vi "V7310.Main.Init.vi"(8 "error in":errorcluster, 11 "Data in":T1={"Status"={"State"=enum."Init", "LaserStatus"=enum."-", "LaserStatusRaw"="", "Ref"=refnum, "RTC TS"=timestamp(0 s since 1904-01-01), "Conn TS"=timestamp(0 s since 1904-01-01), "Msg"=[], "JobInUse"="", "Jobs"=[], "Vars"=[]}, "Sets"={"Address"="192.168.2.1", "Timeout_ms"=5000, "ReconnectPeriod_s"=0, "JobInUse"="", "CoordinatesOffset"={"X"=0.0, "Y"=0.0}}}) -> (0 "error out":errorcluster, 3 "Data out":T1={"Status"={"State"=enum."Init", "LaserStatus"=enum."-", "LaserStatusRaw"="", "Ref"=refnum, "RTC TS"=timestamp(0 s since 1904-01-01), "Conn TS"=timestamp(0 s since 1904-01-01), "Msg"=[], "JobInUse"="", "Jobs"=[], "Vars"=[]}, "Sets"={"Address"="192.168.2.1", "Timeout_ms"=5000, "ReconnectPeriod_s"=0, "JobInUse"="", "CoordinatesOffset"={"X"=0.0, "Y"=0.0}}})   [LabVIEW 2016]
uses:
  V7310.Data.ctl
  V7310.Data.Status.ctl
  V7310.Data.Status.State.ctl
  LowLevel/V7310.LaserStatus.ctl
  LowLevel/V7310.Message.Data.ctl
  LowLevel/V7310.Job.Variable.ctl
  V7310.Data.Sets.ctl
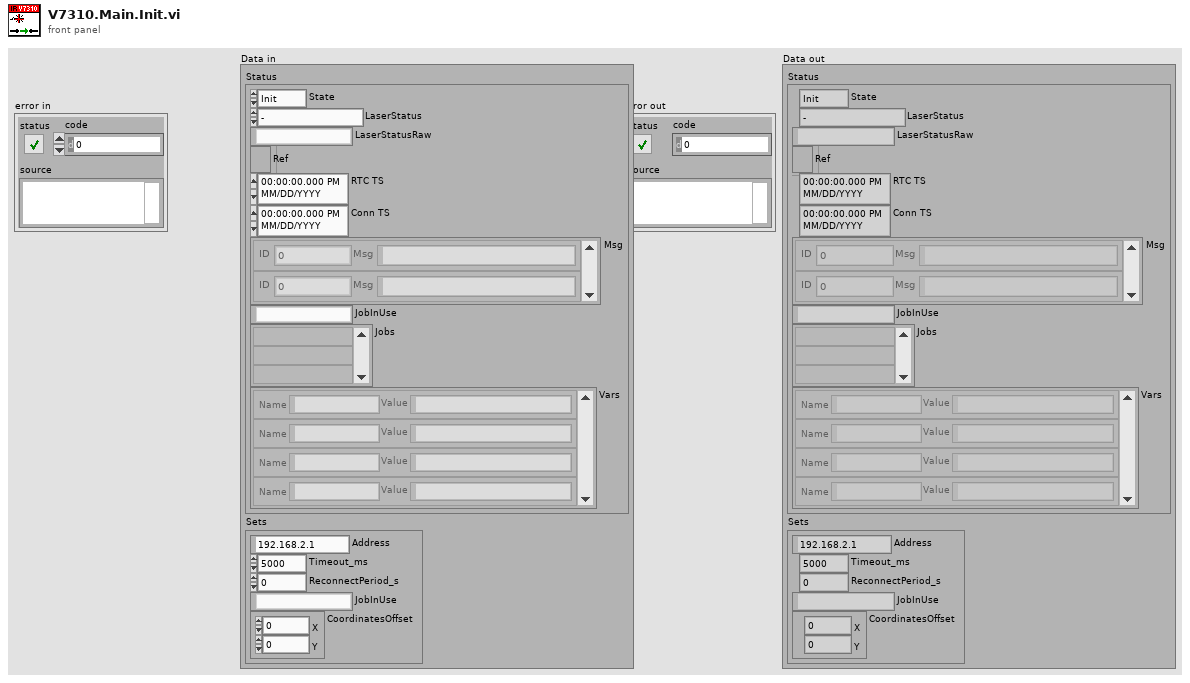
[diagram p1: front panel]
types:
  T1 = typedef "V7310.Data.ctl" = cluster{"Status":T2, "Sets":T7}
  T2 = typedef "V7310.Data.Status.ctl" = cluster{"State":T3, "LaserStatus":T4, "LaserStatusRaw":string, "Ref":refnum<k5>, "RTC TS":timestamp, "Conn TS":timestamp, "Msg":T5[], "JobInUse":string, "Jobs":string[], "Vars":T6[]}
  T3 = typedef "V7310.Data.Status.State.ctl" = enum16{"First", "Init", "Msg", "Error", "Abort", "Idle", "Run"}
  T4 = typedef "V7310.LaserStatus.ctl" = enum16{"-", "FatalError", "Initialize", "KeySwitchOpen", "TimeoutInterlock", "InterlockOpen", "StartUp", "ShutterlockOpen", "Standby", "Ready", "PrepareForMarking", "WaitForTrigger", "Marking"}
  T5 = typedef "V7310.Message.Data.ctl" = cluster{"ID":i32, "Msg":string}
  T6 = typedef "V7310.Job.Variable.ctl" = cluster{"Name":string, "Value":string}
  T7 = typedef "V7310.Data.Sets.ctl" = cluster{"Address":string, "Timeout_ms":i32, "ReconnectPeriod_s":i32, "JobInUse":string, "CoordinatesOffset":cluster{"X":dbl, "Y":dbl}}
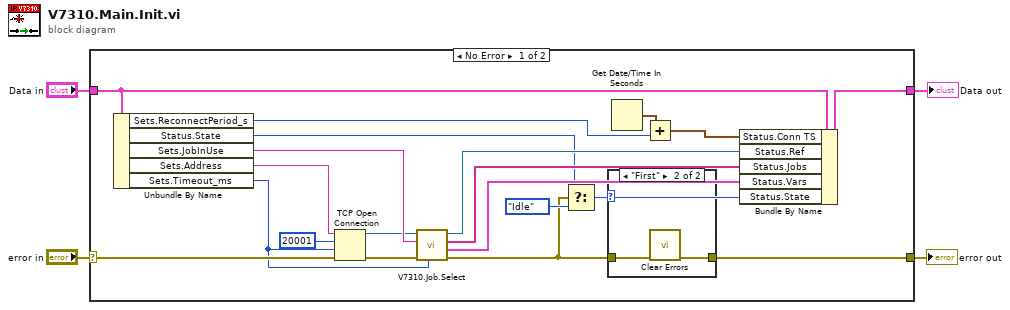
[diagram p0: block diagram]
diagram:
  n1 = case shown="No Error" "error in" {
    selector: "error in" -> [w22 w29]
    tunnel: [w14 w29] -> w3
    tunnel: "Data in" -> [w23 w28]
    tunnel: [w24 w28] -> w1
    frame No Error {
      n2 = Unbundle By Name(w23) -> ("Sets.ReconnectPeriod_s"=w7:i32, "Status.State"=w10:T3, "Sets.JobInUse"=w17:string, "Sets.Address"=w20:string, "Sets.Timeout_ms"=w19:i32)
      n3 = TCP Open Connection(address=w20, remote port or service name=u16 20001, timeout ms (60000)=w19, error in (no error)=w22) -> (connection ID=w6:refnum<k5>, error out=w5:errorcluster)  [unwired: 1 in]
      n4 = call "V7310.Job.Select.vi"("timeout ms (5000)"=w19, "error in"=w5, "Job"=w17, "Connection in"=w6) -> ("error out"=w12:errorcluster, "VarNames"=w15:T6[], "Jobs"=w16:string[], "Connection out"=w18:refnum<k5>)  [unwired: 3 in, 1 out]
      n5 = Select(t=w10, s=w12, f=V7310.Data.Status.State."Idle" ("Status.State")) -> (s? t:f=w11:T3)
      n6 = case shown="\"First\"" w11 {
        tunnel: w12 -> [w25 w27]
        tunnel: [w25 w26] -> w14
        frame Default {
        }
        frame "First" {
          n7 = call <vilib>:"Clear Errors.vi"("error in (no error)"=w27) -> ("error out"=w26:errorcluster)  [unwired: 5 in, 1 out]
        }
      }
      n8 = Get Date/Time In Seconds() -> (seconds since 1Jan1904=w9:timestamp)
      n9 = Add(x=w9, y=w7) -> (x+y=w8:timestamp)
      n10 = Bundle By Name(cluster=w23, "Status.Conn TS"=w8, "Status.Ref"=w18, "Status.Jobs"=w16, "Status.Vars"=w15, "Status.State"=w11) -> (w24:T1)
    }
    frame Error {
    }
  }
  "error out" <- w3
  "Data out" <- w1
